vi "Apply DevInfo to Dev Obj.vi"(8 "error in (no error)":errorcluster, 10 "Dev Obj in":refnum<class "Hardware.lvclass">, 11 "DevInfo in":refnum<class "DevInfo.lvclass">) -> (0 "error out":errorcluster, 2 "Dev Obj out":refnum<class "Hardware.lvclass">, 3 "DevInfo out":refnum<class "DevInfo.lvclass">)   [LabVIEW 2016, in "Hardware.lvlib" / "DevInfo.lvclass"]
uses:
  <userlib>/Common Components/Hardware/DevInfo/DevInfo.lvclass
  <userlib>/Common Components/Hardware/Abstract Hardware/Hardware.lvclass
  <userlib>/Common Components/Hardware/Abstract Hardware/Hardware.lvclass/Hardware.ctl
  <userlib>/Common Components/Hardware/Abstract Hardware/Write DevInfo.vi
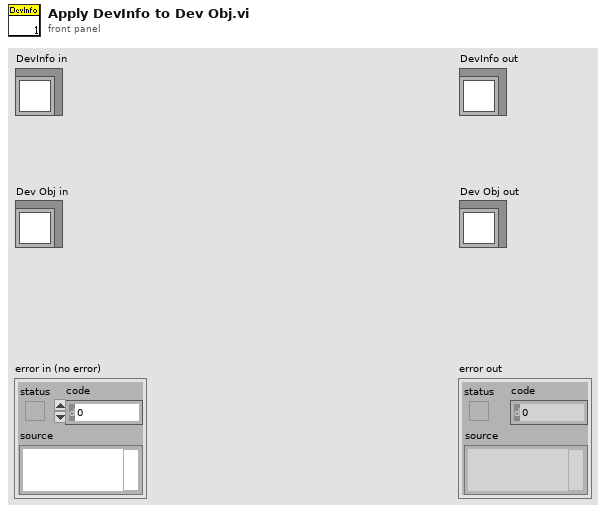
[diagram p1: front panel]
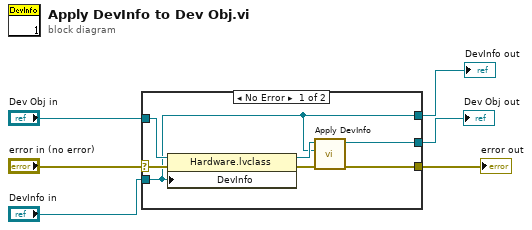
[diagram p0: block diagram]
diagram:
  n1 = case shown="No Error" "error in (no error)" {
    selector: "error in (no error)" -> [w13 w15]
    tunnel: [w8 w15] -> w5
    tunnel: [w10 w14] -> w3
    tunnel: "DevInfo in" -> [w10 w14]
    tunnel: [w7 _] -> w2
    tunnel: "Dev Obj in" -> [w12 _]
    frame No Error {
      n2 = property class="Hardware.lvclass"(reference=w12, error in=w13, "DevInfo"=w10) -> (reference out=w11:refnum<class "Hardware.lvclass">, error out=w9:errorcluster)
      n3 = call-dynamic "Apply DevInfo.vi"("error in (no error)"=w9, "DevInfo"=w10, "Hardware in"=w11) -> ("error out"=w8:errorcluster, "Hardware out"=w7:refnum<class "Hardware.lvclass">)  [unwired: 7 in]
    }
    frame Error {
    }
  }
  "error out" <- w5
  "DevInfo out" <- w3
  "Dev Obj out" <- w2
